vi "Main.vi"() -> ()   [LabVIEW 2020, in "2D Array Example.lvlib"]
uses:
  2D Array Example.lvlib
  2DArrayPanel/2DArrayPanel.lvclass
  OOPanel/2DArrayManager/2DArrayManager.lvclass
  OOPanel/2DArrayManager/2D Index.ctl
  2DArrayPanel2/2DArrayPanel2.lvclass
  C:/dev/lv20CE/lv-oopanel/OOPanel/ArrayPanel/ArrayPanel.lvclass
  C:/dev/lv20CE/lv-oopanel/OOPanel/Panel/Panel.lvclass
  C:/dev/lv20CE/lv-oopanel/Examples/2DArray/2DArrayPanel/2DArrayPanel.lvclass
  C:/dev/lv20CE/lv-oopanel/Examples/2DArray/2DArrayPanel2/2DArrayPanel2.lvclass
panel:
  out "error out":errorcluster
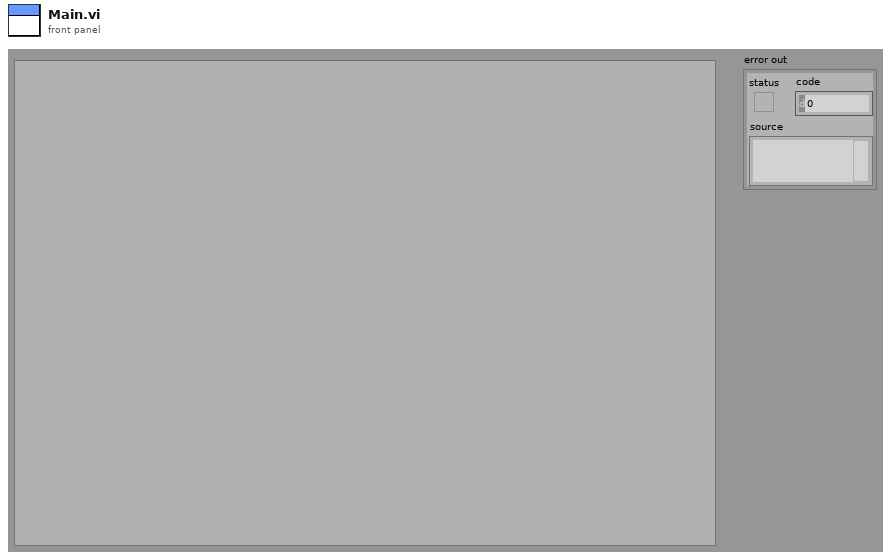
[diagram p1: front panel]
types:
  T1 = typedef "OOPanel.lvlib/2DArrayManager.lvclass/2D Index.ctl" = cluster{"Row":i32, "Col":i32}
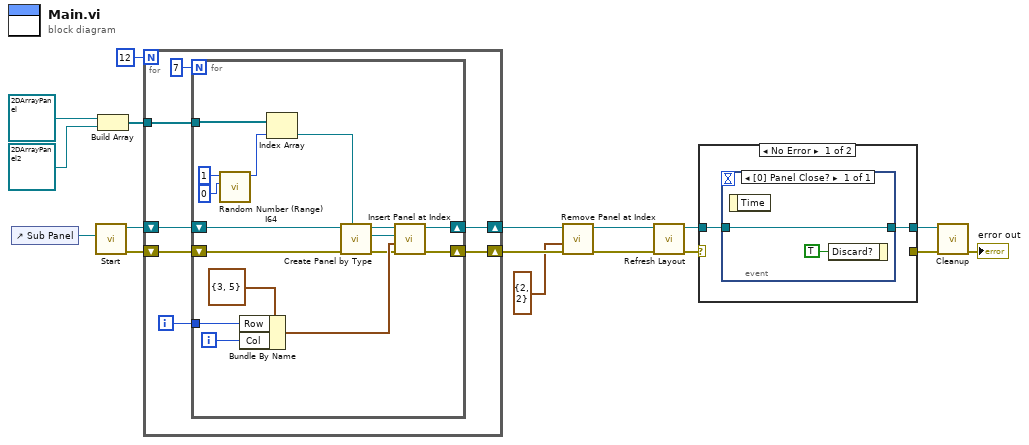
[diagram p0: block diagram]
diagram:
  n1 = control-ref of="Sub Panel"() -> (w16:refnum<vi>)
  n2 = call "Start.vi"("Container"=w16) -> ("error out"=w14:errorcluster, "2DArrayManager out"=w15:refnum<class "2DArrayManager.lvclass">)  [unwired: 9 in]
  n3 = Build Array(refnum<class "2DArrayPanel.lvclass"> refnum ("2D Array Example.lvlib:2DArrayPanel.lvclass"), refnum<class "2DArrayPanel2.lvclass"> refnum ("2D Array Example.lvlib:2DArrayPanel2.lvclass")) -> (w2:refnum<class "ArrayPanel.lvclass">[])
  n4 = for {
    N: 12 -> [_]
    shift-right: [w21] -> w6
    shift-left: w15 -> [w23]
    shift-right: [w19] -> w13
    shift-left: w14 -> [w20]
    tunnel: w2 -> [w18]
    i -> [w22]
    n5 = for {
      N: 7 -> [_]
      tunnel: w22 -> [w34]
      shift-right: [w33] -> w21
      shift-left: w23 -> [w40]
      shift-right: [w30] -> w19
      shift-left: w20 -> [w32]
      tunnel: w18 -> [w27]
      i -> [w35]
      n6 = call <vilib>:"Random Number (Range) I64.vi"("lower bound (-100)"=i64 0 ("upper bound (100)"), "upper bound (100)"=i64 1) -> ("number"=w26:i64)  [unwired: 9 in]
      n7 = Bundle By Name(cluster=T1 {"Row"=3, "Col"=5} ("2D Index"), "Row"=w34, "Col"=w35) -> (w36:T1)
      n8 = Index Array(array=w27, index=w26) -> (element=w25:refnum<class "ArrayPanel.lvclass">)
      n9 = call "Create Panel by Type.vi"("Panel Type"=w25, "error in (no error)"=w32, "2DArrayManager in"=w40) -> ("error out"=w31:errorcluster, "Panel"=w38:refnum<class "ArrayPanel.lvclass">, "2DArrayManager out"=w39:refnum<class "2DArrayManager.lvclass">)  [unwired: 6 in]
      n10 = call "Insert Panel at Index.vi"("error in (no error)"=w31, "2D Index"=w36, "ArrayPanel"=w38, "2DArrayManager in"=w39) -> ("error out"=w30:errorcluster, "2DArrayManager out"=w33:refnum<class "2DArrayManager.lvclass">)  [unwired: 4 in, 2 out]
    }
  }
  n11 = call "Remove Panel at Index.vi"("error in (no error)"=w13, "2D Index"=T1 {"Row"=2, "Col"=2}, "2DArrayManager in"=w6) -> ("error out"=w7:errorcluster, "2DArrayManager out"=w5:refnum<class "2DArrayManager.lvclass">)  [unwired: 5 in, 2 out]
  n12 = call "Refresh Layout.vi"("error in (no error)"=w7, "2DArrayManager in"=w5) -> ("error out"=w10:errorcluster, "2DArrayManager out"=w11:refnum<class "2DArrayManager.lvclass">)  [unwired: 8 in]
  n13 = case shown="No Error" w10 {
    selector: w10 -> [_ w45]
    tunnel: [w42 w46] -> w12
    tunnel: w11 -> [w41 w46]
    tunnel: [_ w45] -> w9
    frame No Error {
      n14 = event shown="[0] Panel Close?" {
        selector: _ -> [_]
        dyn-events: _ -> [_]
        timeout: _ -> [_]
        tunnel: [w43] -> w42
        tunnel: w41 -> [w43]
        event Panel Close? {
          n15 = event-data() -> ()  [unwired: 1 in, 1 out]
          n16 = event-data("Discard?"=TRUE) -> ()  [unwired: 1 in, 1 out]
        }
      }
    }
    frame Error {
    }
  }
  n17 = call "Cleanup.vi"("error in (no error)"=w9, "2DArrayManager in"=w12) -> ("error out"=→"error out":errorcluster)  [unwired: 9 in]
